vi "QRcode Scanner.vi"() -> ()   [LabVIEW 2019]
uses:
  <vilib>/userDefined/High Color/IMAQdx.ctl
  <vilib>/vision/driver/NI_Vision_Acquisition_Software.lvlib
  <vilib>/vision/NI_Vision_Development_Module.lvlib
panel:
  in  "Session In":T1
  out "Data":string
  out "Found ?":bool
  out "Image":T2(plugin-control)
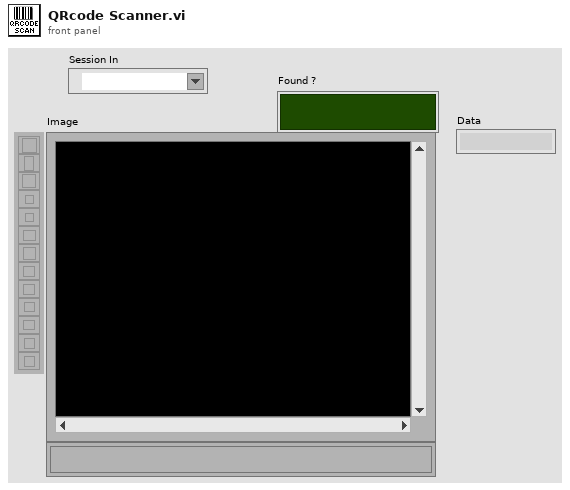
[diagram p1: front panel]
types:
  T1 = typedef "IMAQdx.ctl" = refnum<k21>
  T2 = typedef "IMAQ Image.ctl" = refnum<image>
  T3 = typedef "Image Type" = u32
  T4 = typedef "QR Code Report.ctl" = cluster{"Found?":bool, "Data":string, "Bounding Box":cluster{"x":sgl, "y":sgl}[], "Errors Corrected":u32, "Dimensions (Rows/Cols)":u32, "Version":u32, "QR Model":T5, "Stream Mode":T6, "Barcode Polarity":T7, "Mirrored?":bool, "Append Stream Position":u32, "Size of Append Stream":u32, "First EAN-128 ID":i32, "First Alternate Language ID":i32, "Append Stream ID":u32, "Minimum Edge Strength":u32, "Demodulation Mode":T8, "Cell Sample Size":T9, "Cell Filter Mode":T10}
  T5 = typedef "QR Code Model Type.ctl" = i32
  T6 = typedef "QR Code Stream Mode Type.ctl" = i32
  T7 = typedef "Data Matrix Polarity.ctl" = i32
  T8 = typedef "Demodulation Mode.ctl" = i32
  T9 = typedef "Cell Sample Size.ctl" = i32
  T10 = typedef "Cell Filter Mode.ctl" = i32
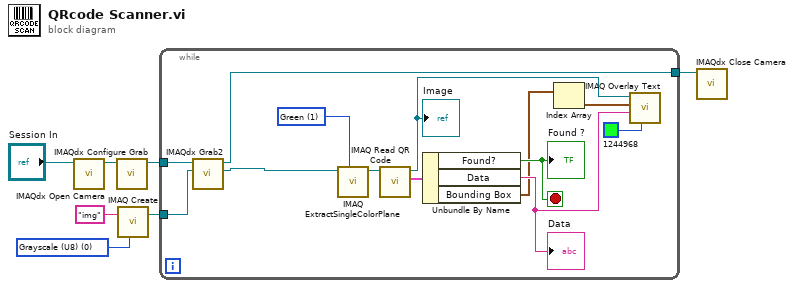
[diagram p0: block diagram]
diagram:
  w1 = T3 0 items=["Grayscale (U8)", "Grayscale (I16)", "Grayscale (SGL)", "Complex (CSG)", "RGB (U32)", "HSL (U32)", "RGB (U64)", "Grayscale (U16)"] ("Image Type")
  n1 = call <vilib>:"IMAQdx Open Camera.vi"("Session In"="Session In") -> ("Session Out"=w7:T1)  [unwired: 9 in, 1 out]
  n2 = call <vilib>:"IMAQdx Configure Grab.vi"("Session In"=w7) -> ("Session Out"=w6:T1)  [unwired: 9 in, 1 out]
  n3 = call "IMAQ Create"("Image Name"="img", "Image Type"=w1) -> ("New Image"=w3:T2)  [unwired: 3 in, 1 out]
  n4 = while {
    tunnel: w6 -> [w20]
    tunnel: [w19] -> w5
    tunnel: w3 -> [w15]
    stop <- w16 stop-if-true
    w14 = 1 items=["Red", "Green", "Blue", "Hue", "Saturation", "Luminance", "Value", "Intensity"] ("Color Plane")
    n5 = call <vilib>:"IMAQdx Grab2.vi"("Image In"=w15, "Session In"=w20) -> ("Image Out"=w18:T2, "Session Out"=w19:T1)  [unwired: 6 in, 2 out]
    n6 = call "IMAQ ExtractSingleColorPlane"("Color Plane"=w14, "Image Src"=w18) -> ("Image Dst Out"=w13:T2)  [unwired: 8 in, 1 out]
    n7 = call "IMAQ Read QR Code"("Image"=w13) -> ("QR Code Report"=w17:T4, "Image (duplicate)"=w9:T2)  [unwired: 7 in, 2 out]
    "Image" <- w9
    n8 = Unbundle By Name(w17) -> ("Found?"=w16:bool, "Data"=w11:string, "Bounding Box"=w8:cluster{"x":sgl, "y":sgl}[])
    "Found ?" <- w16
    "Data" <- w11
    n9 = Index Array(array=w8) -> (element=w12:cluster{"x":sgl, "y":sgl})  [unwired: 1 in]
    n10 = call "IMAQ Overlay Text"("Text Color (black)"=u32 1244968, "String"=w11, "Origin"=w12, "Image"=w9) -> ()  [unwired: 6 in, 2 out]
  }
  n11 = call <vilib>:"IMAQdx Close Camera.vi"("Session In"=w5) -> ()  [unwired: 10 in, 1 out]
